vi "generator.vi"(10 "amplituda":i32, 11 "częstotliwość":i32) -> (0 "error out":errorcluster)   [LabVIEW 2018]
doc: "Ustawia częstotliwość i amplitude na generatorze."
uses:
  Open_device_2017.llb/Select_Instr.ctl
panel:
  out "Open OK (true)":bool
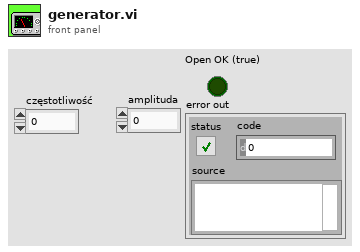
[diagram p1: front panel]
types:
  T1 = typedef "Select_Instr.ctl" = string
  T2 = cluster{"VISA resource name":refnum<visa-resource-name>}
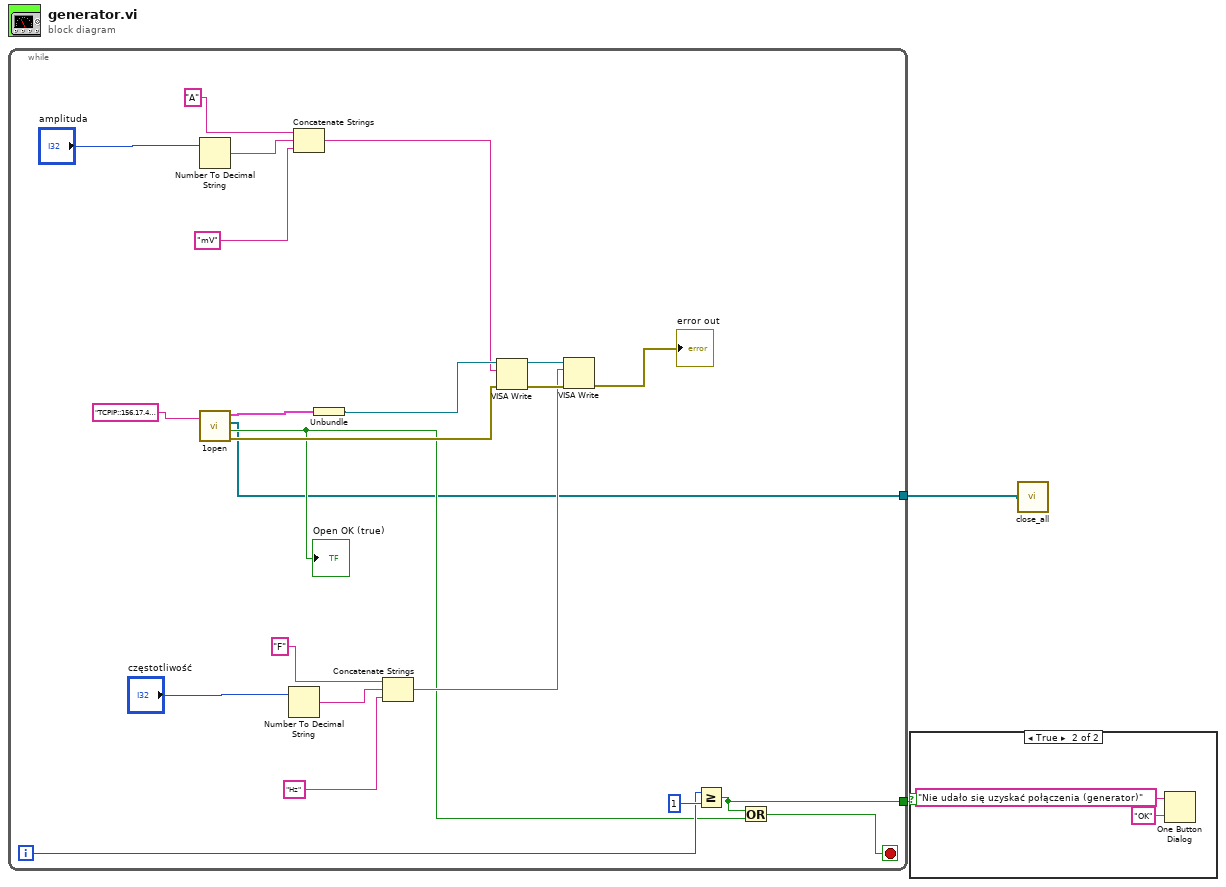
[diagram p0: block diagram]
diagram:
  n1 = while {
    tunnel: [w4] -> w2
    tunnel: [w3] -> w1
    i -> [w6]
    stop <- w7 stop-if-true
    n2 = Number To Decimal String(number="amplituda") -> (decimal integer string=w20:string)  [unwired: 1 in]
    n3 = call "1open.vi"("VISA resource name"=T1 "TCPIP::156.17.45.35::inst26::INSTR" ("Select_Instrument")) -> ("InstrCluster"=w16:T2, "InstrArray"=w3:refnum<visa-resource-name>[], "Open OK (true)"=w5:bool, "error out"=w10:errorcluster)  [unwired: 1 in]
    "Open OK (true)" <- w5
    n4 = Number To Decimal String(number="częstotliwość") -> (decimal integer string=w24:string)  [unwired: 1 in]
    n5 = Concatenate Strings("A", w20, "mV") -> (w14:string)
    n6 = Unbundle(w16) -> ("VISA resource name"=w15:refnum<visa-resource-name>)
    n7 = Concatenate Strings("F", w24, "Hz") -> (w11:string)
    n8 = VISA Write(VISA resource name=w15, write buffer=w14, error in (no error)=w10) -> (VISA resource name out=w13:refnum<visa-resource-name>, error out=w12:errorcluster)  [unwired: 1 out]
    n9 = VISA Write(VISA resource name=w13, write buffer=w11, error in (no error)=w12) -> (error out=→"error out":errorcluster)  [unwired: 2 out]
    n10 = Greater Or Equal?(x=w6, y=1) -> (x >= y?=w4:bool)
    n11 = Or(x=w4, y=w5) -> (x .or. y?=w7:bool)
  }
  n12 = case shown="True" w2 {
    frame False {
    }
    frame True {
      n13 = One Button Dialog(message="Nie udało się uzyskać połączenia (generator)", button name ("OK")="OK") -> ()  [unwired: 1 out]
    }
  }
  n14 = call "close_all.vi"("OpenRes"=w1) -> ()  [unwired: 1 out]
